vi "pause record.vi"(10 "暂停测量":bool, 11 "rec array输入":dbl[][][](array[numeric])) -> (3 "rec array输出":dbl[][][](array[numeric]))   [LabVIEW 2017]
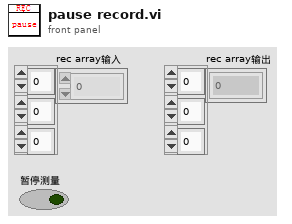
[diagram p1: front panel]
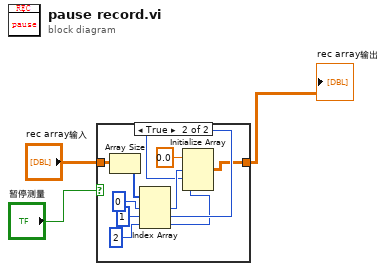
[diagram p0: block diagram]
diagram:
  n1 = case shown="True" "暂停测量" {
    tunnel: "rec array输入" -> [w4 w14]
    tunnel: [w4 w5] -> w2
    frame False {
    }
    frame True {
      n2 = Array Size(array=w14) -> (size(s)=w12:i32[])
      n3 = Index Array(array=w12, index #1=0 ("索引"), index #2=1 ("索引"), index #3=2 ("索引")) -> (element #1=w10:i32, element #2=w8:i32, element #3=w6:i32)
      n4 = Initialize Array(0.0 ("元素"), w10, w8, w6) -> (w5:dbl[][][])
    }
  }
  "rec array输出" <- w2
